vi "PV ActiveLine - FilterTime (TPG362).vi"(7 "W/R":bool, 8 "Fehler (Eingang)":errorcluster, 9 "Sensor 2 Set":i8(ring)=2 items=["Filter off", "Fast", "Normal", "Slow"], 10 "Sensor 1 Set":i8(ring)=2 items=["Filter off", "Fast", "Normal", "Slow"], 11 "Referenz in":refnum<visa-resource-name>) -> (0 "Cluster (Ausgang)":errorcluster, 1 "Sensor 2 Get":i8(ring)=2 items=["Filter off", "fast", "normal", "slow"], 2 "Sensor 1 Get":i8(ring)=2 items=["Filter off", "fast", "normal", "slow"], 3 "Referenz out":refnum<visa-resource-name>)   [LabVIEW 2013, in "PV ActiveLine.lvlib"]
doc: "FIL - Measurement Value Filter\n\nTransmit: FIL [,a,b]\nReceive: a,b\n\nFilter gauge 1,\na =\n0 –> Filter off\n1 –> Fast\n2 –> Normal\n3 –> Slow\n\nFilter gauge 2,\nb =\n0 –> Filter off\n1 –> Fast\n2 –> Normal\n3 –> Slow"
uses:
  C:/Program Files (x86)/National Instruments/LabVIEW 2013/PV ActiveLine/PV ActiveLine.lvlib
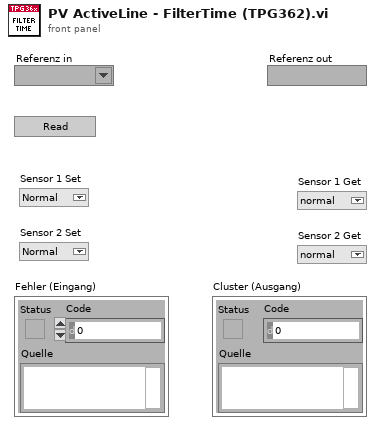
[diagram p1: front panel]
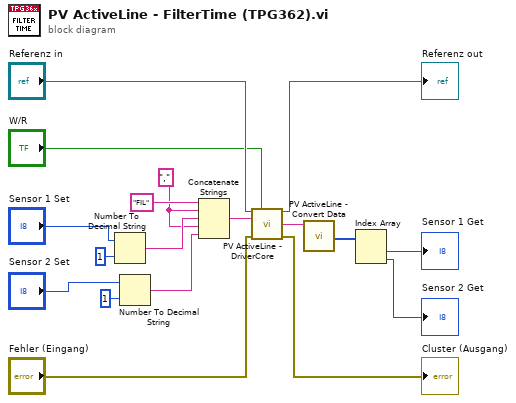
[diagram p0: block diagram]
diagram:
  w14 = "," ("Command")
  n1 = Number To Decimal String(number="Sensor 1 Set", width (-)=i16 1) -> (decimal integer string=w16:string)
  n2 = Number To Decimal String(number="Sensor 2 Set", width (-)=i16 1) -> (decimal integer string=w15:string)
  n3 = Concatenate Strings("FIL" ("Command"), w14, w16, w14, w15) -> (w12:string)
  n4 = call "PV ActiveLine - DriverCore.vi"("Referenz in"="Referenz in", "Write/Read"="W/R", "Command"=w12, "Fehler (Eingang)"="Fehler (Eingang)") -> ("Referenz out"=→"Referenz out":refnum<visa-resource-name>, "String Out"=w4:string, "Cluster (Ausgang)"=→"Cluster (Ausgang)":errorcluster)  [unwired: 9 in]
  n5 = call "PV ActiveLine - Convert Data.vi"("String in"=w4) -> ("Integer Out"=w3:i32[])  [unwired: 7 in, 3 out]
  n6 = Index Array(array=w3) -> (element #1=→"Sensor 1 Get":i32, element #2=→"Sensor 2 Get":i32)  [unwired: 2 in]
